vi "Create Data File.vi"(8 "Error In":errorcluster) -> (0 "Error Out":errorcluster, 3 "File Refnum":refnum<file>)   [LabVIEW 2012]
doc: "This VI performs a series of tasks to create a file for logging data:\n\n1) Check to see if a folder called 'Logged Data' exsists in the same directory as the application\n2) If the folder does not exsist, create it\n3) Create a file name of the format 'Acquired Data <Date> <Time>.txt'\n4) Replace or Create the file"
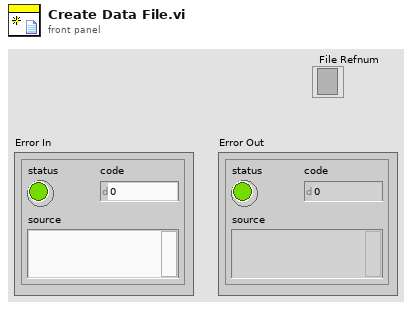
[diagram p1: front panel]
types:
  T1 = enum16{"open", "replace", "create", "open or create", "replace or create", "replace or create with confirmation"}
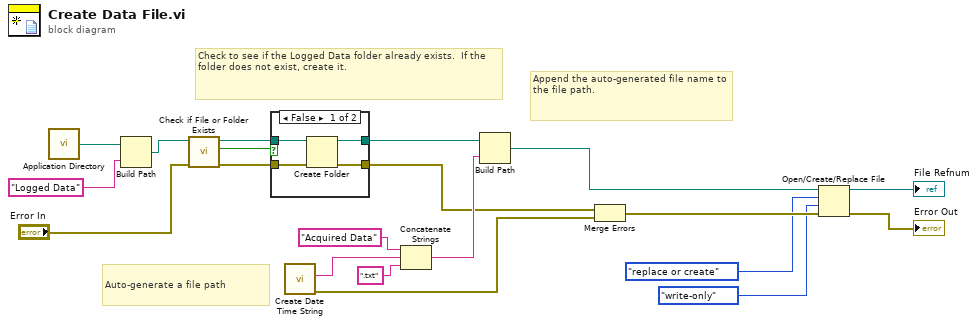
[diagram p0: block diagram]
diagram:
  # "Append the auto-generated file name to the file path."
  # "Check to see if the Logged Data folder already exists.  If the folder does not exist, create it."
  # "Auto-generate a file path"
  n1 = call <vilib>:"Application Directory.vi"() -> ("Application Directory"=w1:path)
  n2 = Build Path(base path=w1, name or relative path="Logged Data" ("prompt (Create Folder)")) -> (appended path=w5:path)
  n3 = call <vilib>:"Check if File or Folder Exists.vi"("error in (no error)"="Error In", "path"=w5) -> ("error out"=w4:errorcluster, "file or folder exists?"=w2:bool, "dup path"=w3:path)  [unwired: 7 in]
  n4 = case shown="False" w2 {
    tunnel: [w24 w26] -> w13
    tunnel: [w23 w25] -> w8
    tunnel: w4 -> [w22 w25]
    tunnel: w3 -> [w21 w26]
    frame False {
      n5 = Create Folder(path (use dialog)=w21, error in=w22) -> (created path=w24:path, error out=w23:errorcluster)  [unwired: 1 in, 1 out]
    }
    frame True {
    }
  }
  n6 = call "Create Date Time String.vi"() -> ("Error Out"=w7:errorcluster, "Date/Time String"=w11:string)  [unwired: 10 in]
  n7 = Concatenate Strings("Acquired Data" ("string"), w11, ".txt" ("string")) -> (w9:string)
  n8 = Build Path(base path=w13, name or relative path=w9) -> (appended path=w20:path)
  n9 = Merge Errors(w8, w7) -> (w19:errorcluster)
  n10 = Open/Create/Replace File(file path (use dialog)=w20, error in=w19, operation (0:open)=T1."replace or create", access (0:read/write)=enum16{"read/write", "read-only", "write-only"}."write-only") -> (refnum out=→"File Refnum":refnum<file>, error out=→"Error Out":errorcluster)  [unwired: 2 in, 1 out]
